vi "rus fit - load data file.vi"(9 "file path":path, 11 "read scan file":T1={"# columns"=3, "create bin file"=TRUE, "do not filter"=FALSE, "normalize phase"=TRUE, "read freq units"=enum."kHz"}) -> (0 "all:max omega":dbl=3099.911666666456, 1 "all:min omega":dbl=450.0, 2 "omega":dbl[](array[numeric]), 3 "x + iy":cdb[](array[numeric]), 4 "file type":enum16{"nothing", "ascii", "binary"}(ring))   [LabVIEW 2015]
uses:
  read scan file control.ctl
  <vilib>/Utility/file.llb/Read From Spreadsheet File (DBL).vi
  <vilib>/Utility/file.llb/Read From Spreadsheet File (string).vi
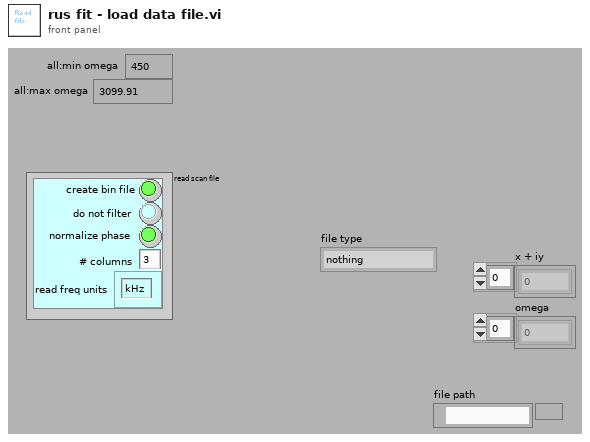
[diagram p1: front panel]
types:
  T1 = typedef "read scan file control.ctl" = cluster{"# columns":i32, "create bin file":bool, "do not filter":bool, "normalize phase":bool, "read freq units":enum16{"kHz", "Hz"}}
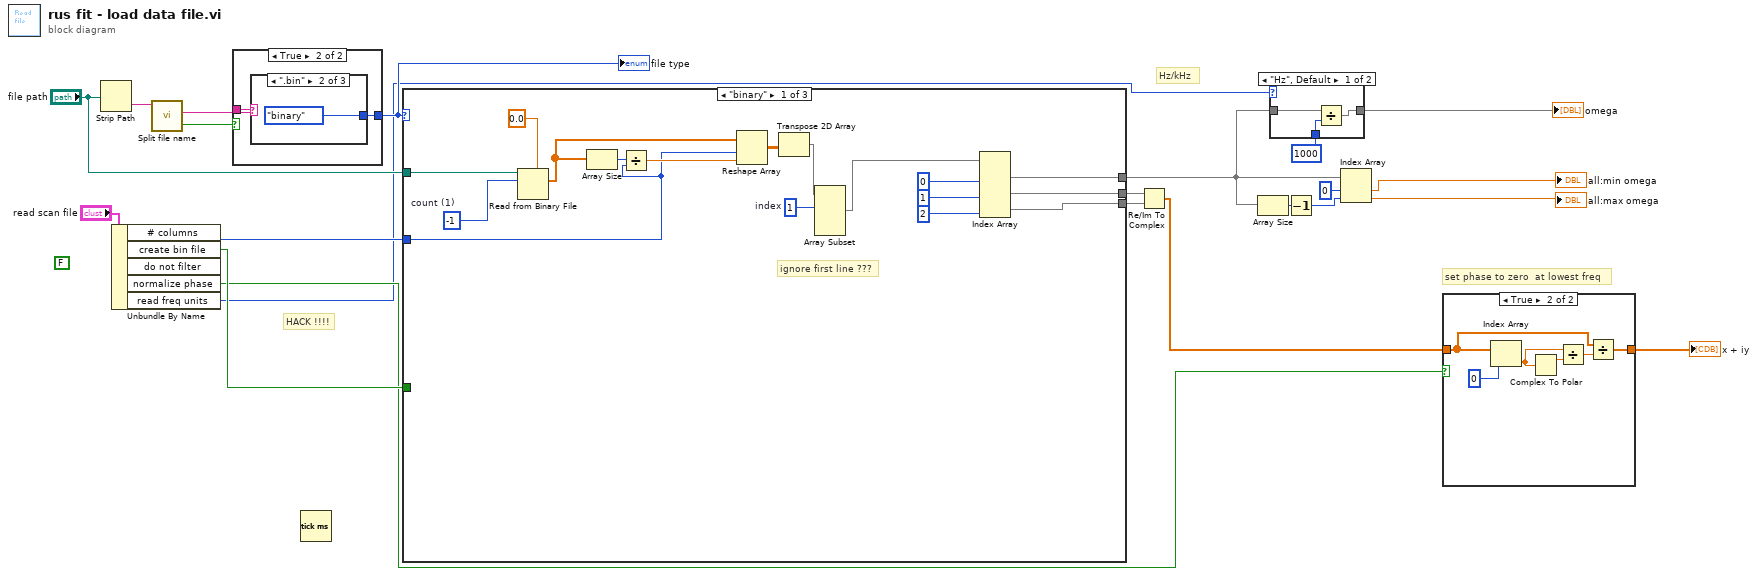
[diagram p0: block diagram]
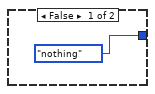
[diagram p3: hidden frame]
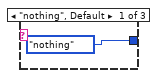
[diagram p4: hidden frame]
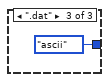
[diagram p5: hidden frame]
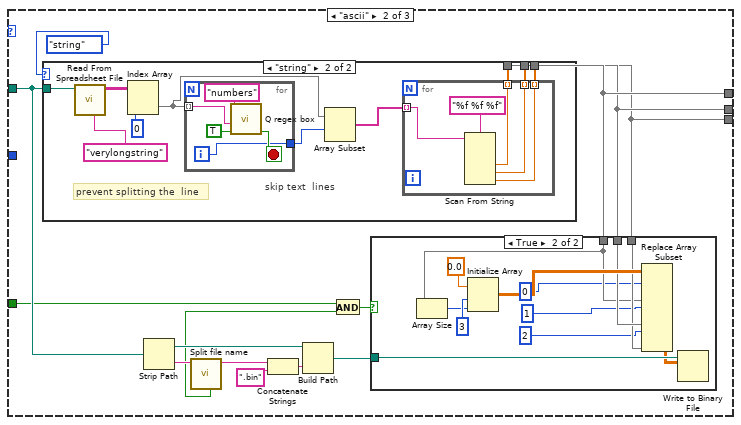
[diagram p6: hidden frame]
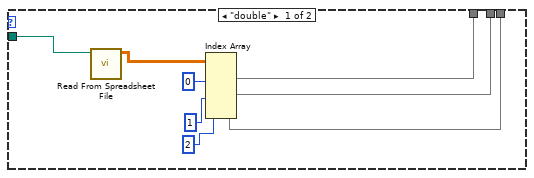
[diagram p8: hidden frame]
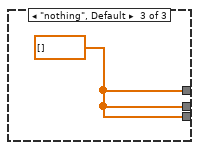
[diagram p9: hidden frame]
diagram:
  (unwired) FALSE ("quote specials")
  # "set phase to zero  at lowest freq"
  # "HACK !!!!"
  # "Hz/kHz"
  n1 = Strip Path(path="file path") -> (name=w18:string)  [unwired: 1 out]
  n2 = Unbundle By Name("read scan file") -> ("# columns"=w4:i32, "create bin file"=w3:bool, "normalize phase"=w2:bool, "read freq units"=w1:enum16{"kHz", "Hz"})  [unwired: 1 out]
  n3 = call "Split file name.vi"("file name"=w18) -> ("extension"=w16:string, "exact match"=w17:bool)  [unwired: 8 in, 1 out]
  n4 = case shown="True" w17 {
    tunnel: w16 -> [_ w25]
    tunnel: [enum16{"nothing", "ascii", "binary"}."nothing" ("action") w24] -> w15
    frame False {
    }
    frame True {
      n5 = case shown="\".bin\"" w25 {
        tunnel: [enum16{"nothing", "ascii", "binary"}."nothing" ("action") enum16{"nothing", "ascii", "binary"}."binary" ("action") enum16{"nothing", "ascii", "binary"}."ascii" ("action")] -> w24
        frame "nothing", Default {
        }
        frame ".bin" {
        }
        frame ".dat" {
        }
      }
    }
  }
  "file type" <- w15
  n6 = Tick Count (ms)() -> ()  [unwired: 1 out]
  n7 = case shown="\"binary\"" w15 {
    tunnel: [w35 w58 w100] -> w8
    tunnel: [w34 w57 w100] -> w21
    tunnel: [w33 w56 w100] -> w20
    tunnel: "file path" -> [w39 w55 _]
    tunnel: w3 -> [_ w46 _]
    tunnel: w4 -> [w29 _ _]
    frame "binary" {
      w32 = 1  # index
      w45 = -1  # count (1)
      # "ignore first line ???"
      n8 = Read from Binary File(5:0.0, 10:w45, 11:w39) -> (2:w42:dbl[])  [unwired: 3 in, 3 out]
      n9 = Array Size(array=w42) -> (size(s)=w41:i32)
      n10 = Divide(x=w41, y=w29) -> (x/y=w40:dbl)
      n11 = Reshape Array(w42, w29, w40) -> (w43:dbl[][])
      n12 = Transpose 2D Array(2D array=w43) -> (transposed array=w31:dbl[][])
      n13 = Array Subset(array=w31, index (row)=w32) -> (w30:dbl[][])  [unwired: 3 in]
      n14 = Index Array(array=w30, index (col) #1=0 ("disabled index (col)"), index (col) #2=1 ("disabled index (col)"), index (col) #3=2 ("disabled index (col)")) -> (element #1=w35:dbl[], element #2=w34:dbl[], element #3=w33:dbl[])  [unwired: 3 in]
    }
    frame "ascii" {
      n15 = case shown="\"string\"" enum16{"double", "string"}."string" {
        tunnel: w55 -> [w79 w89]
        tunnel: [w76 w88] -> w58
        tunnel: [w73 w87] -> w57
        tunnel: [w72 w86] -> w56
        frame "double" {
          n16 = call-poly <vilib>:"Read From Spreadsheet File.vi"("file path (dialog if empty)"=w79) -> ("all rows"=w77:dbl[][])  [unwired: 6 in, 4 out]
          n17 = Index Array(array=w77, index (col) #1=0 ("disabled index (col)"), index (col) #2=1 ("disabled index (col)"), index (col) #3=2 ("disabled index (col)")) -> (element #1=w76:dbl[], element #2=w73:dbl[], element #3=w72:dbl[])  [unwired: 3 in]
        }
        frame "string" {
          # "skip text  lines"
          # "prevent splitting the  line"
          n18 = call-poly <vilib>:"Read From Spreadsheet File.vi"("delimiter (\\t)"="verylongstring" ("delimiter (\\t)"), "file path (dialog if empty)"=w89) -> ("all rows"=w83:string[][])  [unwired: 5 in, 4 out]
          n19 = Index Array(array=w83, index (col)=0 ("index (row)")) -> (element=w81:string[])  [unwired: 1 in]
          n20 = for {
            tunnel: w81 -> [w94] mode=indexing
            tunnel: [w90] -> w80
            i -> [w90]
            stop <- w91 stop-if-true
            n21 = call "Q regex box.vi"("token ?"=TRUE, "string"=w94, "token type"="numbers") -> ("match ?"=w91:bool)  [unwired: 6 in, 2 out]
          }
          n22 = Array Subset(array=w81, index=w80) -> (w82:string[])  [unwired: 1 in]
          n23 = for {
            tunnel: w82 -> [w99] mode=indexing
            tunnel: [w98] -> w88 mode=indexing
            tunnel: [w97] -> w87 mode=indexing
            tunnel: [w96] -> w86 mode=indexing
            n24 = Scan From String(format string="%f %f %f", input string=w99) -> (output 1=w98:dbl, output 2=w97:dbl, output 3=w96:dbl)  [unwired: 5 in, 3 out]
          }
        }
      }
      n25 = Strip Path(path=w55) -> (stripped path=w50:path, name=w54:string)
      n26 = call "Split file name.vi"("file name"=w54) -> ("name"=w53:string, "exact match"=w48:bool)  [unwired: 8 in, 1 out]
      n27 = Concatenate Strings(w53, ".bin" ("string")) -> (w51:string)
      n28 = Build Path(base path=w50, name or relative path=w51) -> (appended path=w49:path)
      n29 = And(x=w46, y=w48) -> (x .and. y?=w47:bool)
      n30 = case shown="True" w47 {
        tunnel: w58 -> [_ w67]
        tunnel: w57 -> [_ w69]
        tunnel: w56 -> [_ w68]
        tunnel: w49 -> [_ w66]
        frame False {
        }
        frame True {
          n31 = Array Size(array=w67) -> (size(s)=w63:i32)
          n32 = Initialize Array(0.0, 3 ("disabled index (col)"), w63) -> (w71:dbl[][])
          n33 = Replace Array Subset(array=w71, new element #1=w67, index (row) #1=0 ("disabled index (col)"), new element #2=w69, index (row) #2=1 ("disabled index (col)"), new element #3=w68, index (row) #3=2 ("disabled index (col)")) -> (w65:dbl[][])  [unwired: 3 in]
          n34 = Write to Binary File(file (use dialog)=w66, data=w65) -> ()  [unwired: 4 in, 3 out]
        }
      }
    }
    frame "nothing", Default {
      w100 = dbl[] [] ("all rows")
    }
  }
  n35 = Re/Im To Complex(1:w20, 2:w21) -> (0:w14:cdb[])
  n36 = Array Size(array=w8) -> (size(s)=w10:i32)
  n37 = case shown="\"Hz\", Default" w1 {
    tunnel: [w102 w104] -> w13
    tunnel: w8 -> [w103 w104]
    tunnel: 1000 ("index") -> [w101 _]
    frame "Hz", Default {
      n38 = Divide(x=w103, y=w101) -> (x/y=w102:dbl[])
    }
    frame "kHz" {
    }
  }
  "omega" <- w13
  n39 = Decrement(x=w10) -> (x-1=w9:i32)
  n40 = Index Array(array=w8, index #1=0 ("index"), index #2=w9) -> (element #1=→"all:min omega":dbl, element #2=→"all:max omega":dbl)
  n41 = case shown="True" w2 {
    tunnel: w14 -> [w105 w107]
    tunnel: [w105 w106] -> w12
    frame False {
    }
    frame True {
      n42 = Index Array(array=w107, index=0) -> (element=w109:cdb)
      n43 = Complex To Polar(r * e^(i*theta)=w109) -> (r=w110:dbl)  [unwired: 1 out]
      n44 = Divide(x=w109, y=w110) -> (x/y=w108:cdb)
      n45 = Divide(x=w107, y=w108) -> (x/y=w106:cdb[])
    }
  }
  "x + iy" <- w12
